vi "AlazarGetWhoTriggeredBySystemHandle.vi"(4 "error in (no error)":errorcluster, 5 "Record Number":u32, 6 "Board ID":u32, 7 "Handle":u64) -> (0 "error out":errorcluster, 2 "Who":u32, 3 "Handle":u64)   [LabVIEW 2009]
doc: "Return which event caused a board system to trigger and capture a record to on-board memory."
uses:
  ATSApi.dll
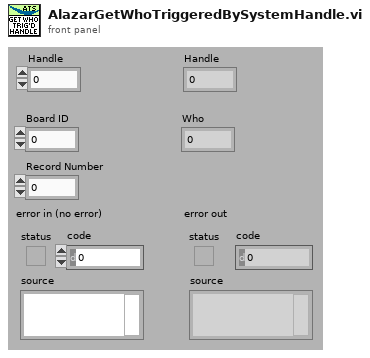
[diagram p1: front panel]
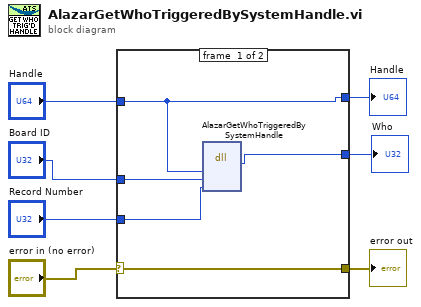
[diagram p0: block diagram]
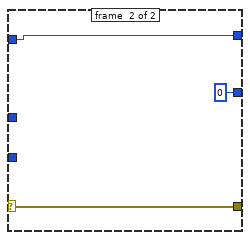
[diagram p2: hidden frame]
diagram:
  n1 = case shown="No Error" "error in (no error)" {
    selector: "error in (no error)" -> [w8 w15]
    tunnel: [w8 w15] -> w6
    tunnel: "Handle" -> [w12 w14]
    tunnel: [w12 w14] -> w4
    tunnel: "Board ID" -> [w11 _]
    tunnel: "Record Number" -> [w10 _]
    tunnel: [w9 0] -> w1
    frame #0 {
      n2 = dll-call lib="ATSApi.dll" fn="AlazarGetWhoTriggeredBySystemHandle"("handle"=w12, "boardID"=w11, "recordNumber"=w10) -> ("return type"=w9:u32)  [unwired: 6 in, 2 out]
    }
    frame #1 {
    }
  }
  "Handle" <- w4
  "error out" <- w6
  "Who" <- w1
